vi "SeCrTs-subvi_quad _L.vi"(10 "input variable":dbl) -> (2 "output variable 2":dbl, 3 "output variable":dbl)   [LabVIEW 2022 SP3]
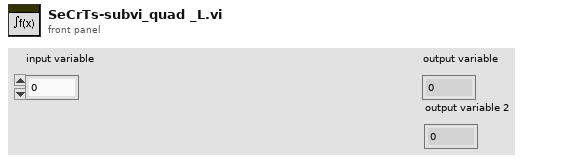
[diagram p1: front panel]
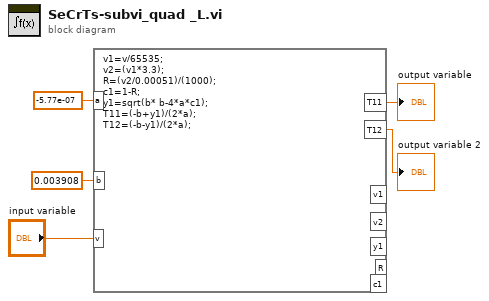
[diagram p0: block diagram]
diagram:
  n1 = formula code="v1=v/65535;\nv2=(v1*3.3);\nR=(v2/0.00051)/(1000);\nc1=1-R;\ny1=sqrt(b* b-4*a*c1);\nT11=(-b+y1)/(2*a);\nT12=(-b-y1)/(2*a);"("a"=-5.77e-07 ("input variable"), "b"=0.003908 ("input variable"), "v"="input variable") -> ("T11"=→"output variable":dbl, "T12"=→"output variable 2":dbl)  [unwired: 5 out]
